vi "lockin - zero amplitude.vi"(6 "measure\noffset?":bool, 8 "error in (no error)":errorcluster, 11 "LockinDAQ":refnum<class "LockinDAQ.lvclass">) -> (0 "error out":errorcluster, 3 "LockinDAQ out":refnum<class "LockinDAQ.lvclass">)   [LabVIEW 2016, in "LockinDAQ.lvclass"]
uses:
  LockinDAQ.lvclass
  LockinDAQ.lvclass/LockinDAQ.ctl
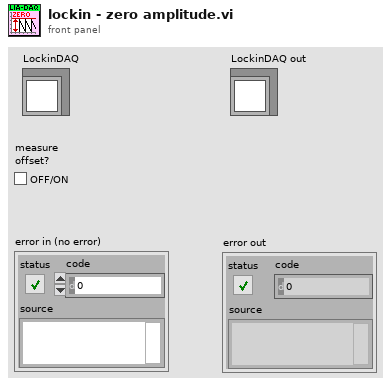
[diagram p1: front panel]
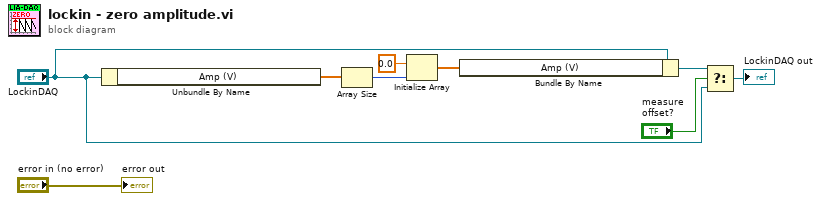
[diagram p0: block diagram]
diagram:
  n1 = Unbundle By Name("LockinDAQ") -> ("Amp (V)"=w7:dbl[])
  n2 = Array Size(array=w7) -> (size(s)=w6:i32)
  n3 = Initialize Array(0.0 ("element"), w6) -> (w9:dbl[])
  n4 = Bundle By Name(cluster="LockinDAQ", "Amp (V)"=w9) -> (w5:refnum<class "LockinDAQ.lvclass">)
  n5 = Select(t=w5, s="measure\noffset?", f="LockinDAQ") -> (s? t:f=→"LockinDAQ out":refnum<class "LockinDAQ.lvclass">)
  "error out" <- "error in (no error)"
